vi "fpga_RefCH Process (P Class_60Hz).vi"(0 "data in <?24.1>":fxp<+/-,24,1>, 5 "Channel number":u8, 7 "Reference index":u8, 9 "input data valid":bool, 12 "ready for output":bool) -> (4 "Filtered Resampling Ref data":fxp<+/-,24,3> format="%.22g", 6 "measured frequency":fxp<+,32,8>, 10 "output valid":bool, 14 "ready for input":bool)   [LabVIEW 2014, in "NI_EP_PMU_FPGA.lvlib"]
uses:
  <vilib>/addons/Electrical Power/PMU/NI_EP_PMU_FPGA.lvlib
  <vilib>/addons/Electrical Power/PQ/Resampling/FPGA/subVIs/fpga_Typedef Fnom.ctl
  <vilib>/rvi/FXPMathLib/basic elements/FxpDiscreteDelay/XNode/nifxpmath_DiscreteDelay.xnode
  <vilib>/addons/Electrical Power/PQ/Resampling/NI_EP_Resample_FPGA.lvlib
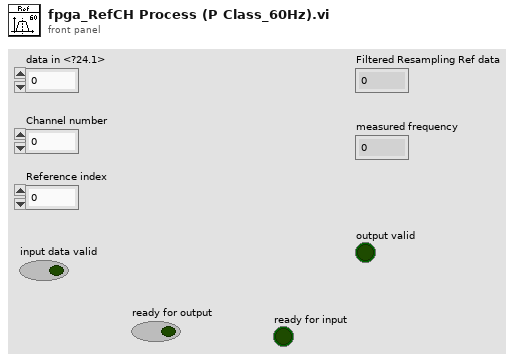
[diagram p1: front panel]
types:
  T1 = typedef "NI_EP_Resample_FPGA.lvlib/fpga_Typedef Fnom.ctl" = u8
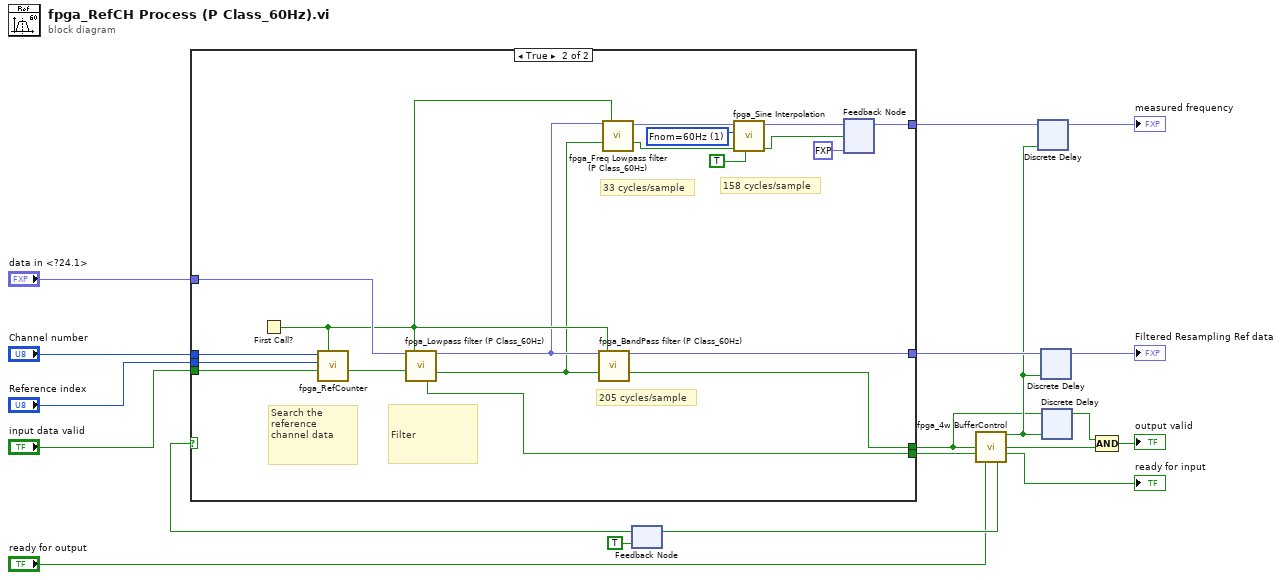
[diagram p0: block diagram]
diagram:
  n1 = feedback #1(TRUE ("logic enable")) -> (w3:bool)
  n2 = case shown="True" w3 {
    tunnel: "input data valid" -> [_ w38]
    tunnel: "Reference index" -> [_ w37]
    tunnel: "Channel number" -> [_ w36]
    tunnel: "data in <?24.1>" -> [_ w35]
    tunnel: [_ w24] -> w15
    tunnel: [_ w22] -> w13
    tunnel: [_ w21] -> w1
    tunnel: [_ w20] -> w6
    frame False {
    }
    frame True {
      w28 = T1 1 items=["Fnom=50Hz", "Fnom=60Hz"] ("Fnom")
      # "158 cycles/sample"
      # "33 cycles/sample"
      # "205 cycles/sample"
      # "Filter"
      # "Search the reference channel data"
      n3 = First Call?() -> (First Call?: T/F=w33:bool)
      n4 = call <vilib>:"fpga_RefCounter.vi"("reset"=w33, "input valid?"=w38, "Reference index"=w37, "NChan"=w36) -> ("Reference channel input valid"=w34:bool)  [unwired: 6 in, 1 out]
      n5 = call <vilib>:"fpga_Lowpass filter (P Class_60Hz).vi"("input data"=w35, "reset"=w33, "input valid"=w34) -> ("output data"=w32:fxp<+/-,24,2>, "output valid"=w31:bool, "ready for input"=w20:bool)  [unwired: 10 in]
      n6 = call <vilib>:"fpga_BandPass filter (P Class_60Hz).vi"("input data"=w32, "reset"=w33, "input valid"=w31) -> ("output data"=w22:fxp<+/-,24,3>, "output valid"=w21:bool)  [unwired: 10 in, 1 out]
      n7 = call <vilib>:"fpga_Freq Lowpass filter (P Class_60Hz).vi"("input data"=w32, "reset"=w33, "input valid"=w31) -> ("output data"=w29:fxp<+/-,24,3>, "output valid"=w30:bool)  [unwired: 10 in, 1 out]
      n8 = call <vilib>:"fpga_Sine Interpolation.vi"("ready for output"=TRUE, "input valid"=w30, "Fnom"=w28, "tach input"=w29) -> ("output valid"=w26:bool, "frequency"=w25:fxp<+,32,8>)  [unwired: 3 in, 3 out]
      n9 = feedback #2(fxp<+,32,8> 60.0 ("frequency")) -> (w24:fxp<+,32,8>)
      n10 = feedback-in #2(w25, w26) -> ()
    }
  }
  n11 = call <vilib>:"fpga_4w BufferControl.vi"("DR"=w1, "RFI"=w6, "RFO"="ready for output") -> ("buff enable"=w12:bool, "output valid"=w10:bool, "ready for input"=→"ready for input":bool, "logic enable"=w4:bool)  [unwired: 9 in]
  n12 = feedback-in #1(w4) -> ()
  n13 = xnode "Discrete Delay"("D"=w15, "enable"=w12) -> ("Q"=→"measured frequency":fxp<+,32,8>)
  n14 = xnode "Discrete Delay"("D"=w13, "enable"=w12) -> ("Q"=→"Filtered Resampling Ref data":fxp<+/-,24,3>)
  n15 = xnode "Discrete Delay"("D"=w1, "enable"=w12) -> ("Q"=w11:bool)
  n16 = Compound Arithmetic op=AND(w11, w10) -> (→"output valid":bool)
